vi "DAQmxTasksVI.vi"(8 "error in (no error)":errorcluster, 10 "ControlQueue":refnum<queue>, 11 "DAQmxTaksContainer_General.lvclass":refnum<class "DAQmxTaksContainer_General.lvclass">) -> ()   [LabVIEW 2015, in "DAQmxTaksContainer_General.lvclass"]
uses:
  DAQmxTaksContainer_General.lvclass
  dependecies/ControlsVIs/Clusters-def/Message types.ctl
  DAQmxTaksContainer_General.lvclass/DAQmxTaksContainer_General.ctl
  GeneralFunctionality/GeneralFunctionality.lvclass/GeneralFunctionality.ctl
  Message/Message.lvclass/Message.ctl
  dependecies/ControlsVIs/Clusters-def/Standard Command.ctl
  DAQmxTask.lvclass
  Message/Message.lvclass
  GeneralFunctionality/GeneralFunctionality.lvclass
panel:
  in  "ReInit":bool
  out "Alarm":bool
  in  "divider":i8(knob)=20 min=1 max=20 step=1 scale=1.0..50.0
  out "ELYSE clock pulses":dbl
  out "Received command":string
  in  "DAQmx Tasks":T1(array[cluster])
  out "error out":errorcluster
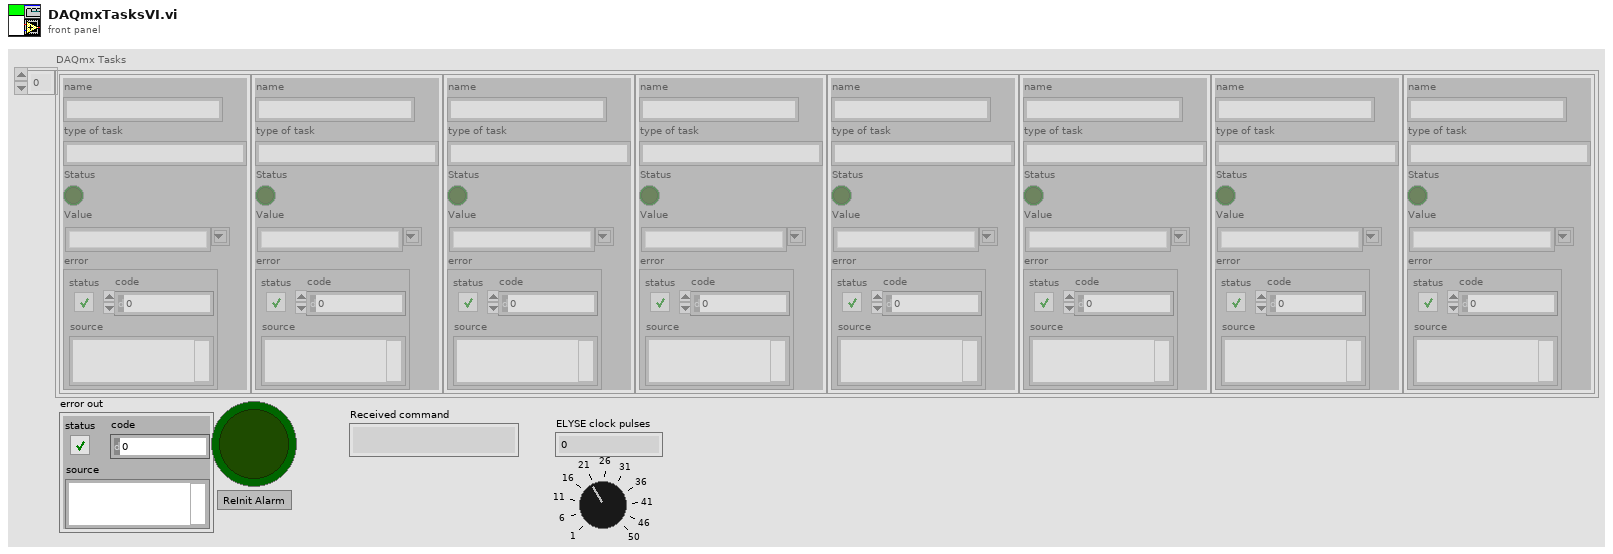
[diagram p1: front panel]
types:
  T1 = cluster{"name":string, "type of task":string, "Status":bool, "Value":string, "error":errorcluster}[]
  T2 = typedef "Message types.ctl" = string
  T3 = typedef "Standard Command.ctl" = cluster{"command":string, "data":variant}
  T4 = cluster{"name":string, "type of task":string, "Status":bool, "Value":string, "error":errorcluster}
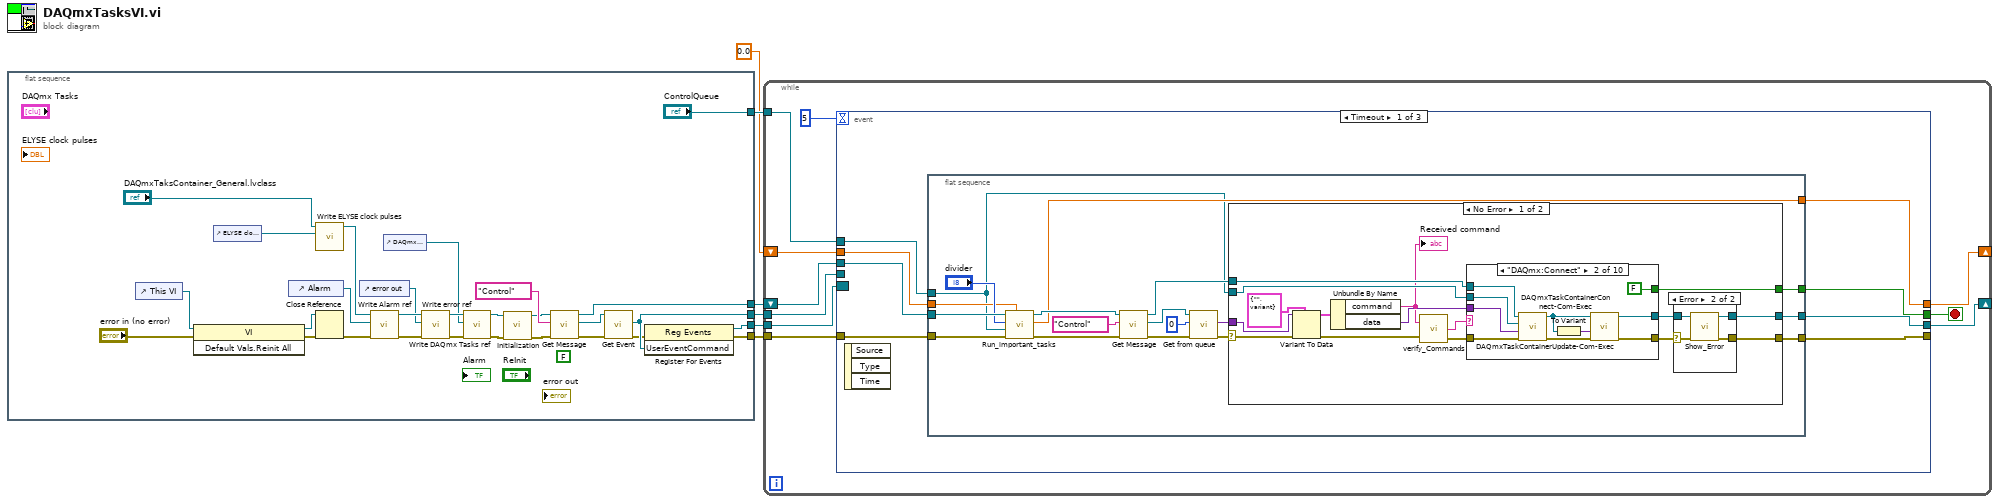
[diagram p0: block diagram]
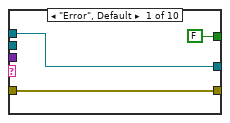
[diagram p3: hidden frame]
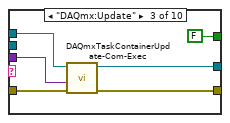
[diagram p4: hidden frame]
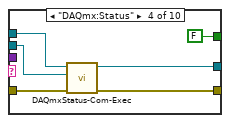
[diagram p5: hidden frame]
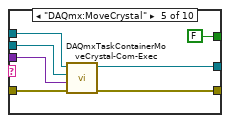
[diagram p6: hidden frame]
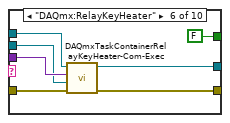
[diagram p7: hidden frame]
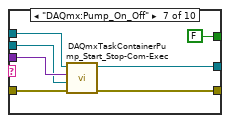
[diagram p8: hidden frame]
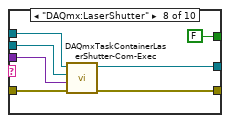
[diagram p9: hidden frame]
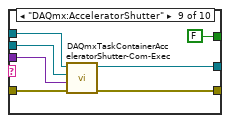
[diagram p10: hidden frame]
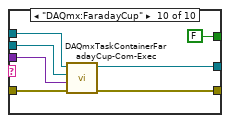
[diagram p11: hidden frame]
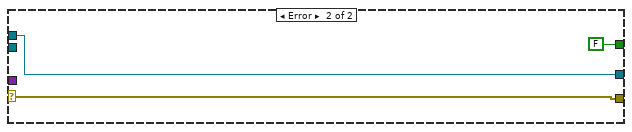
[diagram p12: hidden frame]
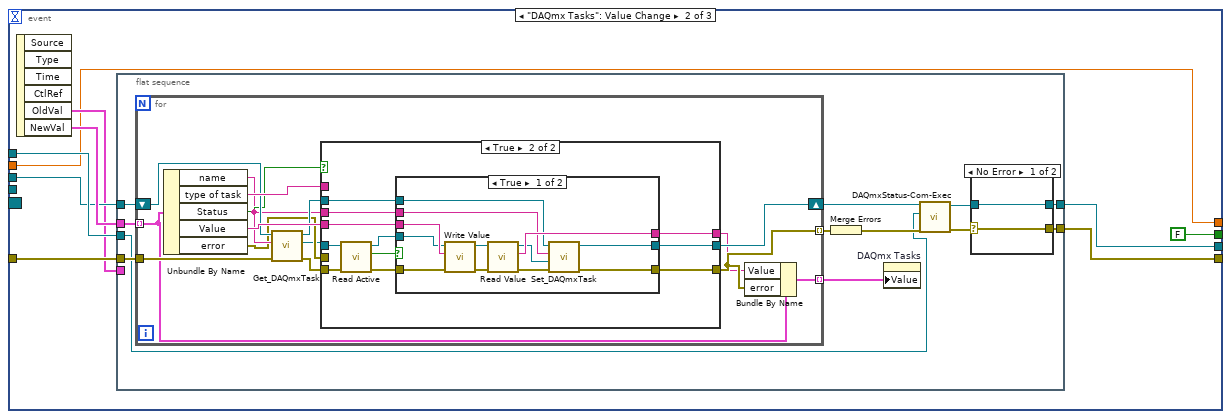
[diagram p13: hidden frame]
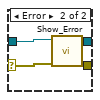
[diagram p14: hidden frame]
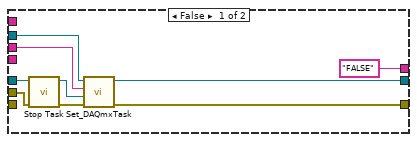
[diagram p15: hidden frame]
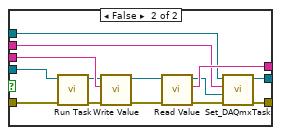
[diagram p16: hidden frame]
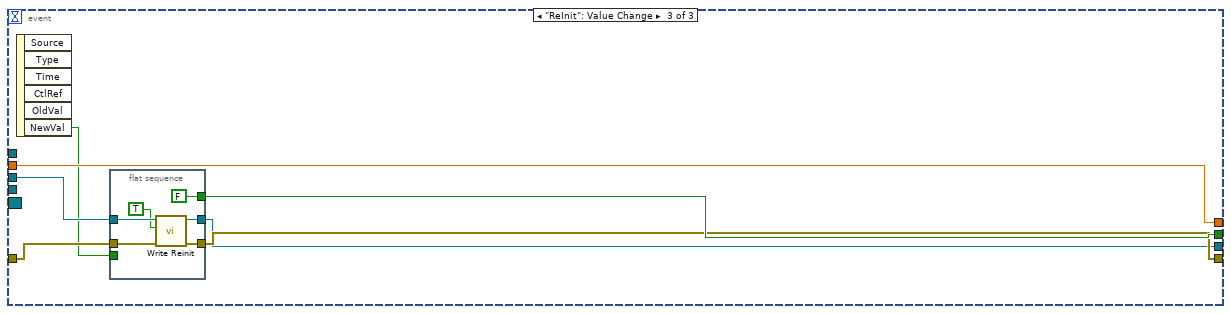
[diagram p17: hidden frame]
diagram:
  n1 = flat-sequence {
    tunnel: [w34] -> w6
    tunnel: [w33] -> w5
    tunnel: ["ControlQueue"] -> w4
    tunnel: [w22] -> w3
    tunnel: [w21] -> w2
    frame #0 {
      (unwired) FALSE ("Clignotant")
      n2 = control-ref of="This VI"() -> (w31:refnum<vi>)
      n3 = invoke class="VI" method="Default Vals.Reinit All"(reference=w31, error in="error in (no error)") -> (reference out=w30:refnum<vi>, error out=w32:errorcluster)  [unwired: 1 in, 1 out]
      n4 = control-ref of="ELYSE clock pulses"() -> (w14:refnum<vi>)
      n5 = control-ref of="Alarm"() -> (w17:refnum<vi>)
      n6 = call "Write ELYSE clock pulses.vi"("ELYSE clock pulses"=w14, "DAQmxTaksContainer_General in"="DAQmxTaksContainer_General.lvclass") -> ("DAQmxTaksContainer_General out"=w16:refnum<class "DAQmxTaksContainer_General.lvclass">)  [unwired: 8 in, 1 out]
      n7 = Close Reference(reference=w30, error in (no error)=w32) -> (error out=w19:errorcluster)
      n8 = control-ref of="error out"() -> (w26:refnum<vi>)
      n9 = call "Write Alarm ref.vi"("error in (no error)"=w19, "Alarm"=w17, "DAQmxTaksContainer_General in"=w16) -> ("error out"=w28:errorcluster, "DAQmxTaksContainer_General out"=w27:refnum<class "DAQmxTaksContainer_General.lvclass">)  [unwired: 7 in]
      n10 = control-ref of="DAQmx Tasks"() -> (w11:refnum<vi>)
      n11 = call "Write error ref.vi"("error in (no error)"=w28, "error"=w26, "GeneralFunctionality in"=w27) -> ("error out"=w12:errorcluster, "GeneralFunctionality out"=w13:refnum<class "DAQmxTaksContainer_General.lvclass">)  [unwired: 7 in]
      n12 = call "Write DAQmx Tasks ref.vi"("error in (no error)"=w12, "DAQmx Tasks ref"=w11, "DAQmxTaksContainer_General in"=w13) -> ("error out"=w8:errorcluster, "DAQmxTaksContainer_General out"=w9:refnum<class "DAQmxTaksContainer_General.lvclass">)  [unwired: 7 in]
      n13 = call-dynamic "Initialization.vi"("error in (no error)"=w8, "DAQmxTaksContainer_General in"=w9) -> ("error out"=w7:errorcluster, "DAQmxTaksContainer_General out"=w10:refnum<class "DAQmxTaksContainer_General.lvclass">)  [unwired: 8 in]
      n14 = call "Get Message.vi"("error in (no error)"=w7, "Message type"=T2 "Control", "GeneralFunctionality en entrée"=w10) -> ("error out"=w24:errorcluster, "Message.lvclass"=w25:refnum<class "Message.lvclass">, "GeneralFunctionality en sortie"=w21:refnum<class "DAQmxTaksContainer_General.lvclass">)  [unwired: 6 in]
      n15 = call "Get Event.vi"("error in (no error)"=w24, "Message en entrée"=w25) -> ("error out"=w18:errorcluster, "UserEventCommand"=w22:refnum<user-event>)  [unwired: 7 in, 1 out]
      n16 = register-events(error in=w18, w22) -> (reference out=w34:refnum<event-registration>, error out=w33:errorcluster)  [unwired: 1 in]
    }
  }
  n17 = while {
    tunnel: w6 -> [w44]
    tunnel: w5 -> [w43]
    shift-right: [w41] -> _
    shift-left: w2 -> [w42]
    tunnel: w4 -> [w40]
    tunnel: w3 -> [w38]
    shift-right: [w35] -> _
    shift-left: 0.0 -> [w36]
    stop <- w37 stop-if-true
    n18 = event shown="[0] Timeout" {
      selector: w44 -> [_ _ _]
      dyn-events: _ -> [_ _ _]
      timeout: 5 -> [_ _ _]
      tunnel: [w47 w168 w254] -> _
      tunnel: w43 -> [w49 w170 w255]
      tunnel: w42 -> [w50 w166 w252]
      tunnel: [w48 w167 w253] -> w41
      tunnel: w40 -> [w51 w169 _]
      tunnel: [w52 FALSE ("NewVal") w257] -> w37
      tunnel: w38 -> [_ _ _]
      tunnel: w36 -> [w46 w163 w256]
      tunnel: [w45 w163 w256] -> w35
      event Timeout {
        n19 = event-data() -> ()  [unwired: 1 in, 3 out]
        n20 = flat-sequence {
          tunnel: [w65] -> w52
          tunnel: [w64] -> w48
          tunnel: [w63] -> w47
          tunnel: w51 -> [w53]
          tunnel: w50 -> [w60]
          tunnel: w49 -> [w58]
          tunnel: w46 -> [w55]
          tunnel: [w54] -> w45
          frame #0 {
            n21 = call "Run_important_tasks.vi"("pulses previous"=w55, "error in (no error)"=w58, "ControlQueue"=w53, "divider"="divider", "DAQmxTaksContainer_General in"=w60) -> ("error out"=w57:errorcluster, "pulses"=w54:dbl, "DAQmxTaksContainer_General out"=w59:refnum<class "DAQmxTaksContainer_General.lvclass">)  [unwired: 4 in]
            n22 = call "Get Message.vi"("error in (no error)"=w57, "Message type"=T2 "Control", "GeneralFunctionality en entrée"=w59) -> ("error out"=w70:errorcluster, "Message.lvclass"=w69:refnum<class "Message.lvclass">, "GeneralFunctionality en sortie"=w61:refnum<class "DAQmxTaksContainer_General.lvclass">)  [unwired: 6 in]
            n23 = call "Get from queue.vi"("error in (no error)"=w70, "timeout in ms (-1)"=0, "Message in"=w69) -> ("error out"=w67:errorcluster, "Data"=w66:variant)  [unwired: 5 in, 2 out]
            n24 = case shown="No Error" w67 {
              selector: w67 -> [w84 w161]
              tunnel: w66 -> [w83 _]
              tunnel: [w78 w161] -> w63
              tunnel: [w82 FALSE] -> w65
              tunnel: [w79 w160] -> w64
              tunnel: w61 -> [w80 w160]
              tunnel: w53 -> [w77 _]
              frame No Error {
                n25 = Variant To Data(error in=w84, type=T3 {"command"="", "data"=variant} ("input cluster"), Variant=w83) -> (data=w86:T3, error out=w75:errorcluster)
                n26 = Unbundle By Name(w86) -> ("command"=w72:string, "data"=w81:variant)
                "Received command" <- w72
                n27 = call "verify_Commands.vi"("Command"=w72, "error in"=w75) -> ("Command out"=w73:string, "error out"=w74:errorcluster)  [unwired: 1 out]
                n28 = case shown="\"DAQmx:Connect\"" w73 {
                  tunnel: w74 -> [w93 w103 w111 w116 w123 w129 w136 w142 w147 w154]
                  tunnel: [w93 w99 w110 w115 w122 w130 w137 w141 w150 w157] -> w71
                  tunnel: [FALSE FALSE FALSE FALSE FALSE FALSE FALSE FALSE FALSE FALSE] -> w82
                  tunnel: [w95 w98 w108 w114 w121 w131 w138 w140 w151 w158] -> w76
                  tunnel: w81 -> [_ w105 w107 _ w124 w128 w135 w143 w148 w155]
                  tunnel: w80 -> [w95 w101 w106 w113 w118 w125 w132 w139 w146 w153]
                  tunnel: w77 -> [_ w104 _ w112 w120 w127 w134 w144 w149 w156]
                  frame "Error", Default {
                  }
                  frame "DAQmx:Connect" {
                    n29 = call "DAQmxTaskContainerConnect-Com-Exec.vi"("error in (no error)"=w103, "data"=w105, "ControlQueue"=w104, "DAQmxTaksContainer_General in"=w101) -> ("error out"=w100:errorcluster, "DAQmxTaksContainer_General out"=w97:refnum<class "DAQmxTaksContainer_General.lvclass">)  [unwired: 6 in]
                    n30 = To Variant(anything=w97) -> (Variant=w96:variant)
                    n31 = call "DAQmxTaskContainerUpdate-Com-Exec.vi"("error in (no error)"=w100, "data"=w96, "DAQmxTaksContainer_General in"=w97) -> ("error out"=w99:errorcluster, "DAQmxTaksContainer_General out"=w98:refnum<class "DAQmxTaksContainer_General.lvclass">)  [unwired: 7 in]
                  }
                  frame "DAQmx:Update" {
                    n32 = call "DAQmxTaskContainerUpdate-Com-Exec.vi"("error in (no error)"=w111, "data"=w107, "DAQmxTaksContainer_General in"=w106) -> ("error out"=w110:errorcluster, "DAQmxTaksContainer_General out"=w108:refnum<class "DAQmxTaksContainer_General.lvclass">)  [unwired: 7 in]
                  }
                  frame "DAQmx:Status" {
                    n33 = call "DAQmxStatus-Com-Exec.vi"("error in (no error)"=w116, "ControlQueue"=w112, "DAQmxTaksContainer_General in"=w113) -> ("error out"=w115:errorcluster, "DAQmxTaksContainer_General out"=w114:refnum<class "DAQmxTaksContainer_General.lvclass">)  [unwired: 7 in]
                  }
                  frame "DAQmx:MoveCrystal" {
                    n34 = call "DAQmxTaskContainerMoveCrystal-Com-Exec.vi"("error in (no error)"=w123, "data"=w124, "ControlQueue"=w120, "DAQmxTaksContainer_General in"=w118) -> ("error out"=w122:errorcluster, "DAQmxTaksContainer_General out"=w121:refnum<class "DAQmxTaksContainer_General.lvclass">)  [unwired: 6 in]
                  }
                  frame "DAQmx:RelayKeyHeater" {
                    n35 = call "DAQmxTaskContainerRelayKeyHeater-Com-Exec.vi"("error in (no error)"=w129, "ControlQueue"=w127, "data"=w128, "DAQmxTaksContainer_General in"=w125) -> ("error out"=w130:errorcluster, "DAQmxTaksContainer_General out"=w131:refnum<class "DAQmxTaksContainer_General.lvclass">)  [unwired: 6 in]
                  }
                  frame "DAQmx:Pump_On_Off" {
                    n36 = call "DAQmxTaskContainerPump_Start_Stop-Com-Exec.vi"("error in (no error)"=w136, "ControlQueue"=w134, "data"=w135, "DAQmxTaksContainer_General in"=w132) -> ("error out"=w137:errorcluster, "DAQmxTaksContainer_General out"=w138:refnum<class "DAQmxTaksContainer_General.lvclass">)  [unwired: 6 in]
                  }
                  frame "DAQmx:LaserShutter" {
                    n37 = call "DAQmxTaskContainerLaserShutter-Com-Exec.vi"("error in (no error)"=w142, "data"=w143, "ControlQueue"=w144, "DAQmxTaksContainer_General in"=w139) -> ("error out"=w141:errorcluster, "DAQmxTaksContainer_General out"=w140:refnum<class "DAQmxTaksContainer_General.lvclass">)  [unwired: 6 in]
                  }
                  frame "DAQmx:AcceleratorShutter" {
                    n38 = call "DAQmxTaskContainerAcceleratorShutter-Com-Exec.vi"("error in (no error)"=w147, "data"=w148, "ControlQueue"=w149, "DAQmxTaksContainer_General in"=w146) -> ("error out"=w150:errorcluster, "DAQmxTaksContainer_General out"=w151:refnum<class "DAQmxTaksContainer_General.lvclass">)  [unwired: 6 in]
                  }
                  frame "DAQmx:FaradayCup" {
                    n39 = call "DAQmxTaskContainerFaradayCup-Com-Exec.vi"("error in (no error)"=w154, "data"=w155, "ControlQueue"=w156, "DAQmxTaksContainer_General in"=w153) -> ("error out"=w157:errorcluster, "DAQmxTaksContainer_General out"=w158:refnum<class "DAQmxTaksContainer_General.lvclass">)  [unwired: 6 in]
                  }
                }
                n40 = case shown="Error" w71 {
                  selector: w71 -> [w87 w89]
                  tunnel: [w88 w92] -> w79
                  tunnel: [w87 w91] -> w78
                  tunnel: w76 -> [w88 w90]
                  frame No Error {
                  }
                  frame Error {
                    n41 = call "Show_Error.vi"("error in (no error)"=w89, "DAQmxTaksContainer_General in"=w90) -> ("error out"=w91:errorcluster, "DAQmxTaksContainer_General out"=w92:refnum<class "DAQmxTaksContainer_General.lvclass">)  [unwired: 8 in]
                  }
                }
              }
              frame Error {
              }
            }
          }
        }
      }
      event "DAQmx Tasks": Value Change {
        n42 = event-data() -> ("OldVal"=w165:T1, "NewVal"=w171:T1)  [unwired: 1 in, 4 out]
        n43 = flat-sequence {
          tunnel: w171 -> [w183]
          tunnel: w170 -> [w182]
          tunnel: w169 -> [w172]
          tunnel: [w178] -> w168
          tunnel: [w179] -> w167
          tunnel: w166 -> [w180]
          tunnel: w165 -> [_]
          frame #0 {
            n44 = for {
              tunnel: w183 -> [w195] mode=indexing
              tunnel: w182 -> [w201]
              tunnel: [w193] -> w181 mode=indexing
              shift-right: [w197] -> w175
              shift-left: w180 -> [w202]
              tunnel: [w194] -> w177 mode=indexing
              n45 = Unbundle By Name(w195) -> ("name"=w198:string, "type of task"=w204:string, "Status"=w200:bool, "Value"=w203:string, "error"=w196:errorcluster)
              n46 = call "Get_DAQmxTask.vi"("error in (no error)"=w201, "Task name"=w198, "DAQmxTaksContainer_General in"=w202) -> ("error out"=w190:errorcluster, "DAQmx Task"=w191:refnum<class "DAQmxTask.lvclass">, "DAQmxTaksContainer_General out"=w199:refnum<class "DAQmxTaksContainer_General.lvclass">)  [unwired: 6 in]
              n47 = case shown="True" w200 {
                tunnel: w204 -> [_ _]
                tunnel: w203 -> [_ w223]
                tunnel: w196 -> [w213 _]
                tunnel: w199 -> [w211 w215]
                tunnel: w198 -> [w212 w214]
                tunnel: [w210 w216] -> w197
                tunnel: [w209 w222] -> w193
                tunnel: ["FALSE" ("Result") w224] -> w192
                tunnel: w191 -> [w208 w221]
                tunnel: w190 -> [_ w220]
                frame False {
                  n48 = call "Stop Task.vi"("error in (no error)"=w213, "DAQmxTask in"=w208) -> ("error out"=w205:errorcluster, "DAQmxTask out"=w206:refnum<class "DAQmxTask.lvclass">)  [unwired: 8 in]
                  n49 = call "Set_DAQmxTask.vi"("error in (no error)"=w205, "DAQmxTask"=w206, "Task name"=w212, "DAQmxTaksContainer_General in"=w211) -> ("error out"=w209:errorcluster, "DAQmxTaksContainer_General out"=w210:refnum<class "DAQmxTaksContainer_General.lvclass">)  [unwired: 6 in]
                }
                frame True {
                  n50 = call-dynamic "Read Active.vi"("error in (no error)"=w220, "DAQmxTask in"=w221) -> ("error out"=w218:errorcluster, "Active?"=w219:bool, "DAQmxTask out"=w217:refnum<class "DAQmxTask.lvclass">)  [unwired: 7 in]
                  n51 = case shown="True" w219 {
                    tunnel: [w234 w248] -> w224
                    tunnel: w223 -> [w233 w247]
                    tunnel: [w230 w241] -> w222
                    tunnel: w218 -> [w232 w246]
                    tunnel: w217 -> [w231 w245]
                    tunnel: [w229 w240] -> w216
                    tunnel: w215 -> [w227 w239]
                    tunnel: w214 -> [w226 w237]
                    frame True {
                      n52 = call-dynamic "Write Value.vi"("error in (no error)"=w232, "Data"=w233, "DAQmxTask en entrée"=w231) -> ("error out"=w236:errorcluster, "DAQmxTask en sortie"=w235:refnum<class "DAQmxTask.lvclass">)  [unwired: 7 in]
                      n53 = call-dynamic "Read Value.vi"("error in (no error)"=w236, "DAQmxTask en entrée"=w235) -> ("error out"=w225:errorcluster, "Data string"=w234:string, "DAQmxTask en sortie"=w228:refnum<class "DAQmxTask.lvclass">)  [unwired: 6 in, 1 out]
                      n54 = call "Set_DAQmxTask.vi"("error in (no error)"=w225, "DAQmxTask"=w228, "Task name"=w226, "DAQmxTaksContainer_General in"=w227) -> ("error out"=w230:errorcluster, "DAQmxTaksContainer_General out"=w229:refnum<class "DAQmxTaksContainer_General.lvclass">)  [unwired: 6 in]
                    }
                    frame False {
                      n55 = call "Run Task.vi"("error in (no error)"=w246, "DAQmxTask in"=w245) -> ("error out"=w243:errorcluster, "DAQmxTask out"=w244:refnum<class "DAQmxTask.lvclass">)  [unwired: 8 in]
                      n56 = call-dynamic "Write Value.vi"("error in (no error)"=w243, "Data"=w247, "DAQmxTask en entrée"=w244) -> ("error out"=w250:errorcluster, "DAQmxTask en sortie"=w249:refnum<class "DAQmxTask.lvclass">)  [unwired: 7 in]
                      n57 = call-dynamic "Read Value.vi"("error in (no error)"=w250, "DAQmxTask en entrée"=w249) -> ("error out"=w242:errorcluster, "Data string"=w248:string, "DAQmxTask en sortie"=w238:refnum<class "DAQmxTask.lvclass">)  [unwired: 6 in, 1 out]
                      n58 = call "Set_DAQmxTask.vi"("error in (no error)"=w242, "DAQmxTask"=w238, "Task name"=w237, "DAQmxTaksContainer_General in"=w239) -> ("error out"=w241:errorcluster, "DAQmxTaksContainer_General out"=w240:refnum<class "DAQmxTaksContainer_General.lvclass">)  [unwired: 6 in]
                    }
                  }
                }
              }
              n59 = Bundle By Name(cluster=w195, "Value"=w192, "error"=w193) -> (w194:T4)
            }
            n60 = Merge Errors(w181) -> (w176:errorcluster)
            n61 = property on="DAQmx Tasks" class="Arr (strict)"("Value"=w177) -> ()  [unwired: 2 in, 2 out]
            n62 = call "DAQmxStatus-Com-Exec.vi"("error in (no error)"=w176, "ControlQueue"=w172, "DAQmxTaksContainer_General in"=w175) -> ("error out"=w173:errorcluster, "DAQmxTaksContainer_General out"=w174:refnum<class "DAQmxTaksContainer_General.lvclass">)  [unwired: 7 in]
            n63 = case shown="No Error" w173 {
              selector: w173 -> [w184 w186]
              tunnel: [w185 w189] -> w179
              tunnel: [w184 w188] -> w178
              tunnel: w174 -> [w185 w187]
              frame No Error {
              }
              frame Error {
                n64 = call "Show_Error.vi"("error in (no error)"=w186, "DAQmxTaksContainer_General in"=w187) -> ("error out"=w188:errorcluster, "DAQmxTaksContainer_General out"=w189:refnum<class "DAQmxTaksContainer_General.lvclass">)  [unwired: 8 in]
              }
            }
          }
        }
      }
      event "ReInit": Value Change {
        n65 = event-data() -> ("NewVal"=w251:bool)  [unwired: 1 in, 5 out]
        n66 = flat-sequence {
          tunnel: [FALSE ("NewVal")] -> w257
          tunnel: w255 -> [w262]
          tunnel: [w261] -> w254
          tunnel: [w260] -> w253
          tunnel: w252 -> [w259]
          tunnel: w251 -> [_]
          frame #0 {
            n67 = call "Write Reinit.vi"("error in (no error)"=w262, "Reinit"=TRUE ("AlarmOccured"), "DAQmxTaksContainer_General in"=w259) -> ("error out"=w261:errorcluster, "DAQmxTaksContainer_General out"=w260:refnum<class "DAQmxTaksContainer_General.lvclass">)  [unwired: 7 in]
          }
        }
      }
    }
  }
